vi "Page.Back.vi"(8 "error in (no error)":errorcluster, 11 "State Variables":T1) -> (0 "error out":errorcluster, 3 "State Variables":T1)   [LabVIEW 2015]
uses:
  Types/Main.StateVariables.ctl
  <vilib>/Utility/miscctls.llb/LVPositionTypeDef.ctl
  Types/Execute.UserEventRefs.ctl
  <vilib>/NI Veristand/Execution/Workspace/SystemStateRegEventRef.ctl
  <vilib>/NI Veristand/Execution/Workspace/Target State Info.ctl
  <vilib>/NI Veristand/Execution/Workspace/Target State.ctl
  <vilib>/NI Veristand/Execution/WaveformStreaming/Waveform Data Watcher Event Data (DBL).ctl
  <vilib>/NI Veristand/Execution/WaveformStreaming/WaveformStreamSpecification.ctl
  NationalInstruments.VeriStand.ClientAPI
  <vilib>/NI Veristand/Execution/Workspace/SystemStateEventRef.ctl
  <vilib>/NI Veristand/Execution/Workspace/WorkspaceAPI.ctl
  Types/UI.Object.ctl
  Types/Waveforms.Info.ctl
  <vilib>/NI Veristand/Execution/WaveformStreaming/Registered Waveform Streams Data Event Refnum (DBL).ctl
  <vilib>/NI Veristand/Execution/WaveformStreaming/WaveformDataWatcherDBL.ctl
  <vilib>/NI Veristand/Execution/WaveformStreaming/WaveformStreamingAPI.ctl
  <vilib>/NI Veristand/Execution/Workspace/NI_VS Workspace ExecutionAPI.lvlib
  <vilib>/NI Veristand/Execution/WaveformStreaming/NI_VS Waveform Streaming Interface.lvlib
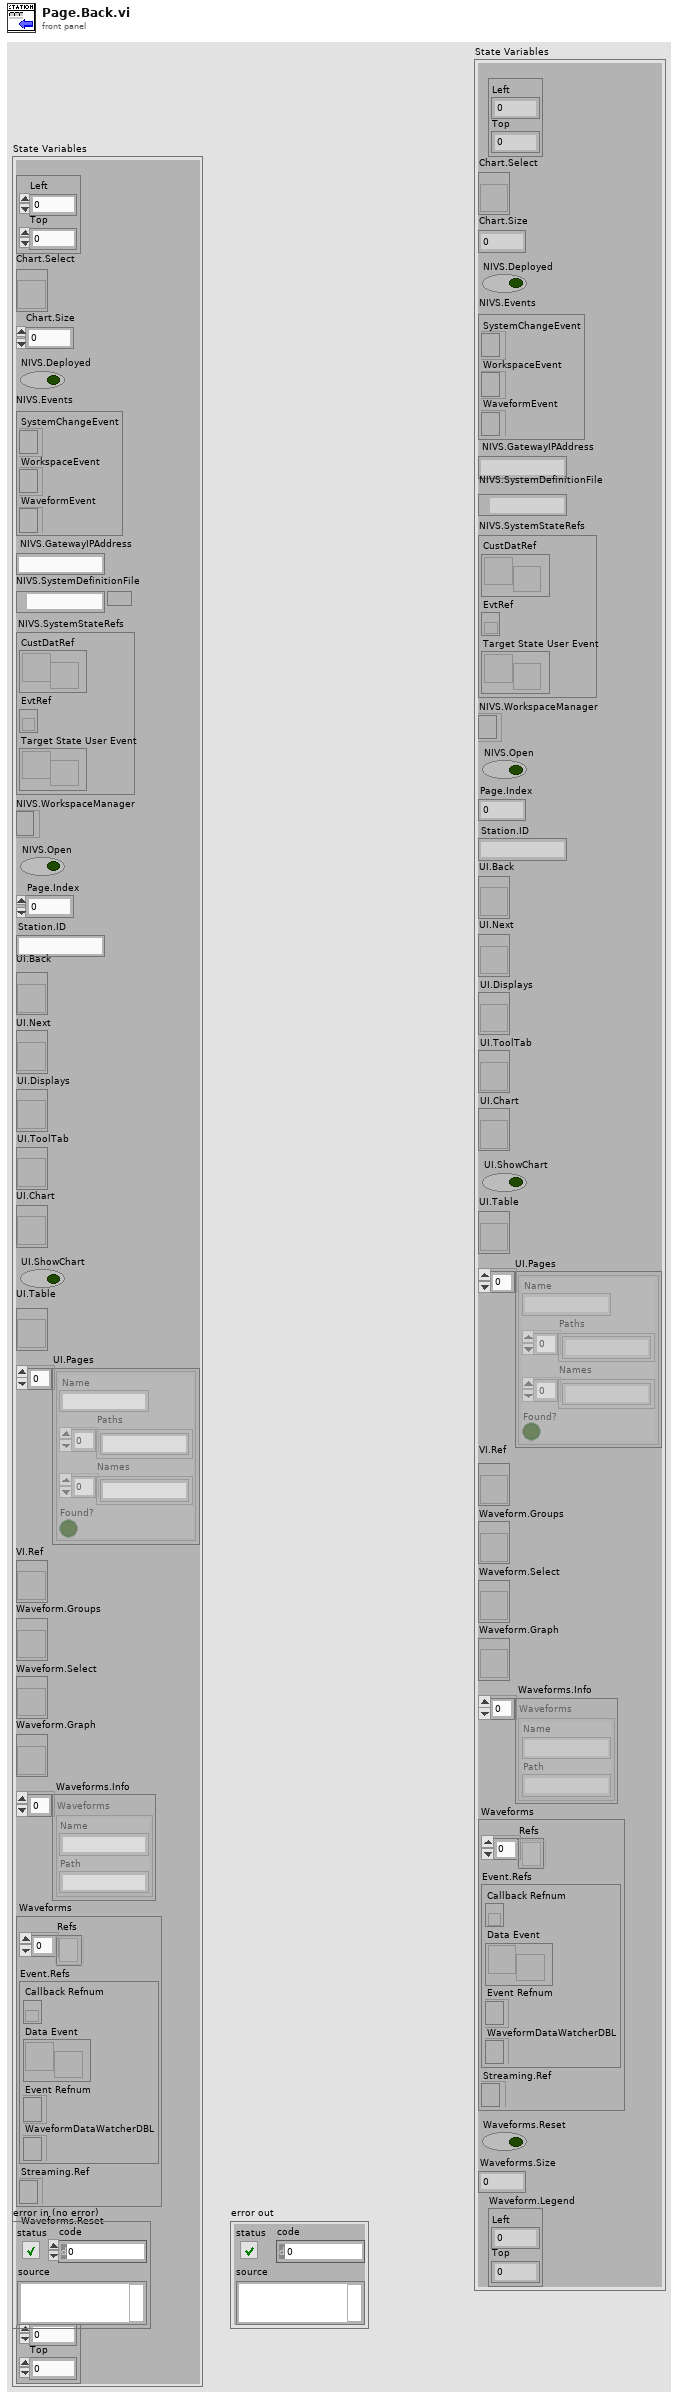
[diagram p1: front panel]
types:
  T1 = typedef "Main.StateVariables.ctl" = cluster{"Chart.Legend":T2, "Chart.Select":refnum<vi>, "Chart.Size":i32, "NIVS.Deployed":bool, "NIVS.Events":T3, "NIVS.GatewayIPAddress":string, "NIVS.SystemDefinitionFile":path, "NIVS.SystemStateRefs":T5, "NIVS.WorkspaceManager":T6, "NIVS.Open":bool, "Page.Index":u32, "Station.ID":string, "UI.Back":refnum<vi>, "UI.Next":refnum<vi>, "UI.Displays":refnum<vi>, "UI.ToolTab":refnum<vi>, "UI.Chart":refnum<vi>, "UI.ShowChart":bool, "UI.Table":refnum<vi>, "UI.Pages":T7[], "VI.Ref":refnum<vi>, "Waveform.Groups":refnum<vi>, "Waveform.Select":refnum<vi>, "Waveform.Graph":refnum<vi>, "Waveforms.Info":T8[], "Waveforms":cluster{"Refs":T9[], "Event.Refs":T10, "Streaming.Ref":T12}, "Waveforms.Reset":bool, "Waveforms.Size":i32, "Waveform.Legend":T2}
  T2 = typedef "LVPositionTypeDef.ctl" = cluster{"Left":i32, "Top":i32}
  T3 = typedef "Execute.UserEventRefs.ctl" = cluster{"SystemChangeEvent":T4, "WorkspaceEvent":refnum<event-registration>, "WaveformEvent":refnum<event-registration>}
  T4 = typedef "NI_VS Workspace ExecutionAPI.lvlib/SystemStateRegEventRef.ctl" = refnum<event-registration>
  T5 = typedef "NI_VS Workspace ExecutionAPI.lvlib/SystemStateEventRef.ctl" = cluster{"CustDatRef":refnum<user-event>, "EvtRef":refnum<k27>, "Target State User Event":refnum<user-event>}
  T6 = typedef "NI_VS Workspace ExecutionAPI.lvlib/WorkspaceAPI.ctl" = refnum<k24>
  T7 = typedef "UI.Object.ctl" = cluster{"Name":string, "Paths":string[], "Names":string[], "Found?":bool}
  T8 = typedef "Waveforms.Info.ctl" = cluster{"Name":string, "Path":string}
  T9 = typedef "NI_VS Waveform Streaming Interface.lvlib/WaveformStreamSpecification.ctl" = refnum<k24>
  T10 = typedef "NI_VS Waveform Streaming Interface.lvlib/Registered Waveform Streams Data Event Refnum (DBL).ctl" = cluster{"Callback Refnum":refnum<k27>, "Data Event":refnum<user-event>, "Event Refnum":refnum<event-registration>, "WaveformDataWatcherDBL":T11}
  T11 = typedef "NI_VS Waveform Streaming Interface.lvlib/WaveformDataWatcherDBL.ctl" = refnum<k24>
  T12 = typedef "NI_VS Waveform Streaming Interface.lvlib/WaveformStreamingAPI.ctl" = refnum<k24>
  T13 = enum8{"Enabled", "Disabled", "Disabled and Grayed Out"}
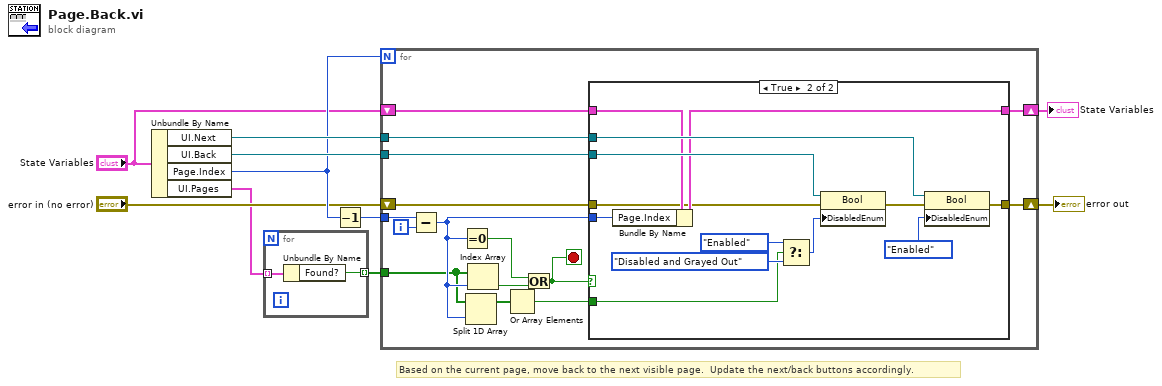
[diagram p0: block diagram]
diagram:
  # "Based on the current page, move back to the next visible page.  Update the next/back buttons accordingly."
  n1 = Unbundle By Name("State Variables") -> ("UI.Next"=w9:refnum<vi>, "UI.Back"=w8:refnum<vi>, "Page.Index"=w6:u32, "UI.Pages"=w1:T7[])
  n2 = for {
    tunnel: [w12] -> w2 mode=indexing
    tunnel: w1 -> [w11] mode=indexing
    n3 = Unbundle By Name(w11) -> ("Found?"=w12:bool)
  }
  n4 = Decrement(x=w6) -> (x-1=w7:u32)
  n5 = for {
    N: w6 -> [_]
    tunnel: w7 -> [w27]
    tunnel: w9 -> [w24]
    tunnel: w8 -> [w23]
    tunnel: w2 -> [w18]
    shift-right: [w25] -> w10
    shift-left: "error in (no error)" -> [w26]
    shift-right: [w13] -> w3
    shift-left: "State Variables" -> [w14]
    i -> [w20]
    stop <- w15 stop-if-true
    n6 = Subtract(x=w27, y=w20) -> (x-y=w19:u32)
    n7 = Equal To 0?(x=w19) -> (x = 0?=w22:bool)
    n8 = Split 1D Array(array=w18, index=w19) -> (first subarray=w17:bool[])  [unwired: 1 out]
    n9 = Index Array(array=w18, index=w19) -> (element=w21:bool)
    n10 = Or Array Elements(Boolean array=w17) -> (logical OR=w16:bool)
    n11 = Or(x=w22, y=w21) -> (x .or. y?=w15:bool)
    n12 = case shown="True" w15 {
      tunnel: w23 -> [_ w42]
      tunnel: w24 -> [_ w37]
      tunnel: [w29 w35] -> w25
      tunnel: w26 -> [w29 w30]
      tunnel: w19 -> [_ w32]
      tunnel: w16 -> [_ w34]
      tunnel: w14 -> [w28 w33]
      tunnel: [w28 w31] -> w13
      frame False {
      }
      frame True {
        n13 = Bundle By Name(cluster=w33, "Page.Index"=w32) -> (w31:T1)
        n14 = Select(t=T13."Enabled" ("Disabled"), s=w34, f=T13."Disabled and Grayed Out") -> (s? t:f=w39:T13)
        n15 = property class="Bool"(reference=w42, error in=w30, "DisabledEnum"=w39) -> (error out=w38:errorcluster)  [unwired: 1 out]
        n16 = property class="Bool"(reference=w37, error in=w38, "DisabledEnum"=T13."Enabled" ("Disabled")) -> (error out=w35:errorcluster)  [unwired: 1 out]
      }
    }
  }
  "error out" <- w10
  "State Variables" <- w3
